vi "Equi-Ripple BandStop (DBL).vi"(0 "X":dbl[](array[numeric]), 1 "lower pass freq":dbl=0.2 format="%0.2f", 3 "# of taps":i32=33, 4 "lower stop freq":dbl=0.25000000000000006 format="%0.2f", 5 "higher pass freq":dbl=0.4000000000000001 format="%0.2f", 8 "higher stop freq":dbl=0.3500000000000001 format="%0.2f", 9 "sampling freq: fs":dbl=1.0 format="%0.2f") -> (6 "Filtered X":dbl[](array[numeric]), 7 "error":i32)   [LabVIEW 2014, in "NI_AALBase.lvlib"]
doc: "Generates a bandstop FIR digital filter with equi-ripple characteristics using the Parks-McClellan algorithm and <B>higher pass freq</B>, <B>lower pass freq</B>, <B># of taps</B>, <B>lower stop freq</B>, <B>higher stop freq</B>, and <B>sampling freq: fs</B>. The Equi-Ripple BandStop VI then applies a linear-phase, bandstop filter to the input sequence <B>X</B> using the Convolution VI to obtain <B>Filtered X</B>. Wire data to the <B>X</B> input to determine the polymorphic instance to use or manually select the instance."
uses:
  NI_AALBase.lvlib
  1D Convolution (DBL).vi
  NI_AALPro.lvlib
panel:
  # "Equi-Ripple\n BandStop FIR Filter"
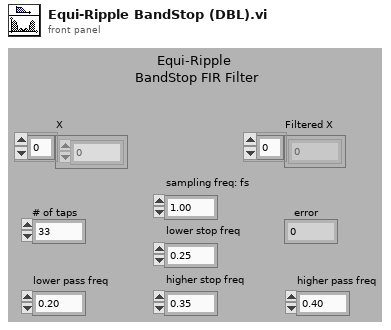
[diagram p1: front panel]
types:
  T1 = cluster{"Amplitude":dbl, "DC":dbl, "lower pass freq":dbl, "Weight":dbl}
  T2 = cluster{"Amplitude":dbl, "lower stop freq":dbl, "higher stop freq":dbl, "Weight":dbl}
  T3 = cluster{"Amplitude":dbl, "higher pass freq":dbl, dbl, "Weight":dbl}
  T4 = cluster{"Amplitude":dbl, "higher pass freq":dbl, "higher stop freq":dbl, "Weight":dbl}[]
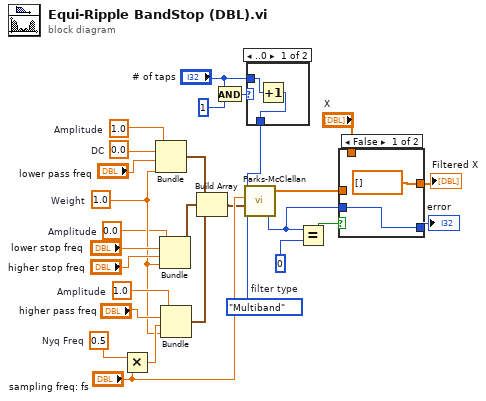
[diagram p0: block diagram]
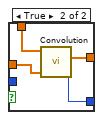
[diagram p3: hidden frame]
diagram:
  w10 = enum32{"Multiband", "Differentiator", "Hilbert"}."Multiband"  # filter type
  w5 = 1.0  # Amplitude
  w26 = 0.5  # Nyq Freq
  w3 = 0.0  # Amplitude
  w4 = 1.0  # Weight
  w2 = 0.0  # DC
  w1 = 1.0  # Amplitude
  n1 = Multiply(x=w26, y="sampling freq: fs") -> (x*y=w15:dbl)
  n2 = Bundle("Amplitude"=w1, "DC"=w2, "lower pass freq"="lower pass freq", "Weight"=w4) -> (w25:T1)  [unwired: 1 in]
  n3 = Bundle("Amplitude"=w3, "lower stop freq"="lower stop freq", "higher stop freq"="higher stop freq", "Weight"=w4) -> (w24:T2)  [unwired: 1 in]
  n4 = Bundle("Amplitude"=w5, "higher pass freq"="higher pass freq", w15, "Weight"=w4) -> (w14:T3)  [unwired: 1 in]
  n5 = Build Array(w25, w24, w14) -> (w11:T4)
  n6 = And(x="# of taps", y=1) -> (x .and. y?=w19:i32)
  n7 = case shown="..0" w19 {
    tunnel: "# of taps" -> [w30 w31]
    tunnel: [w29 w31] -> w13
    frame ..0 {
      n8 = Increment(x=w30) -> (x+1=w29:i32)
    }
    frame 1.. {
    }
  }
  n9 = call "Parks-McClellan.vi"("filter type"=w10, "Band Parameters"=w11, "sampling freq: fs"="sampling freq: fs", "# of taps"=w13) -> ("error"=w7:i32, "h"=w9:dbl[])  [unwired: 1 out]
  n10 = Equal?(x=w7, y=0) -> (x = y?=w8:bool)
  n11 = case shown="False" w8 {
    tunnel: w7 -> [w33 _]
    tunnel: [w33 w34] -> w23
    tunnel: [dbl[] [] ("empty array") w35] -> w22
    tunnel: "X" -> [_ w37]
    tunnel: w9 -> [_ w36]
    frame False {
    }
    frame True {
      n12 = call-poly "Convolution.vi"("Y"=w36, "X"=w37) -> ("error"=w34:i32, "X * Y"=w35:dbl[])  [unwired: 8 in]
    }
  }
  "Filtered X" <- w22
  "error" <- w23
